vi "AG SubNavUtil.vi"(7 "Progress Ref":refnum<vi>, 8 "error out":errorcluster, 9 "AG SubNav Colors":T1={"On Tab Background"=14869218, "Off Tab Background"=12763842, "Text On Color"=5395026, "Text Off Color"=16777225}, 10 "NewVal":i32, 11 "Tab Ref":refnum<vi>) -> (0 "error IO":errorcluster)   [LabVIEW 2012]
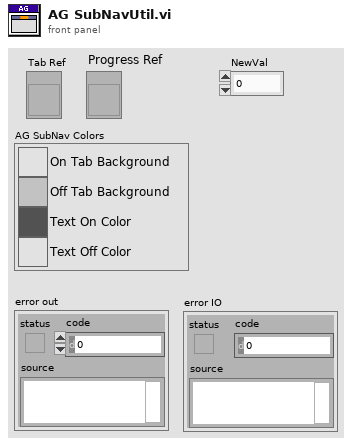
[diagram p1: front panel]
types:
  T1 = cluster{"On Tab Background":u32, "Off Tab Background":u32, "Text On Color":u32, "Text Off Color":u32}
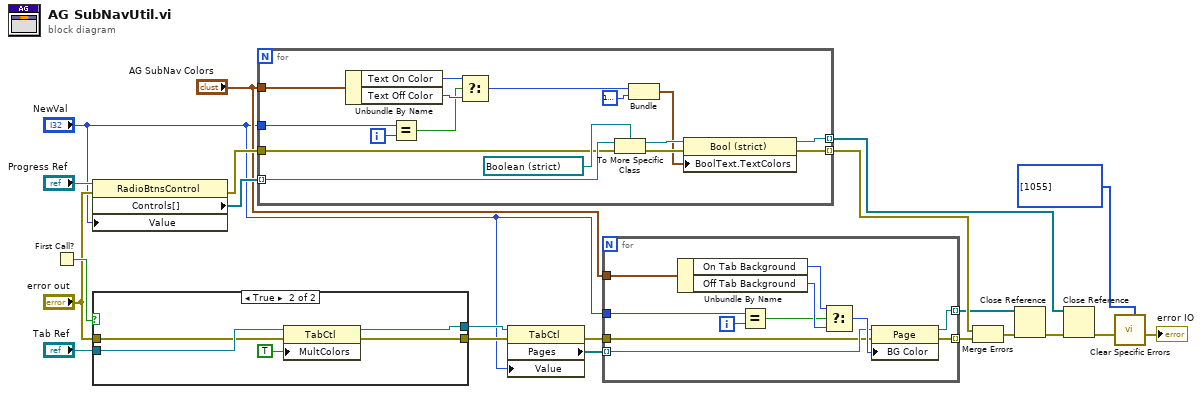
[diagram p0: block diagram]
diagram:
  n1 = First Call?() -> (First Call?: T/F=w20:bool)
  n2 = property class="RadioBtnsControl"(reference="Progress Ref", error in="error out", "Value"="NewVal") -> (error out=w15:errorcluster, "Controls[]"=w16:refnum<vi>[])  [unwired: 1 out]
  n3 = case shown="True" w20 {
    tunnel: "Tab Ref" -> [w22 w28]
    tunnel: "error out" -> [w23 w27]
    tunnel: [w23 w26] -> w19
    tunnel: [w22 w25] -> w18
    frame False {
    }
    frame True {
      n4 = property on="Property Node" class="TabCtl"(reference=w28, error in=w27, "MultColors"=TRUE ("Allow Multiple Colors")) -> (reference out=w25:refnum<vi>, error out=w26:errorcluster)
    }
  }
  n5 = for {
    tunnel: "NewVal" -> [w43]
    tunnel: w16 -> [w39] mode=indexing
    tunnel: "AG SubNav Colors" -> [w40]
    tunnel: w15 -> [w31]
    tunnel: [w30] -> w13 mode=indexing
    tunnel: [w29] -> w9 mode=indexing
    i -> [w44]
    n6 = Unbundle By Name(w40) -> ("Text On Color"=w35:u32, "Text Off Color"=w34:u32)
    n7 = Equal?(x=w43, y=w44) -> (x = y?=w33:bool)
    n8 = Select(t=w35, s=w33, f=w34) -> (s? t:f=w32:u32)
    n9 = To More Specific Class(target class=refnum<vi> refnum ("Radio Selection 1"), reference=w39, error in=w31) -> (specific class reference=w42:refnum<vi>, error out=w38:errorcluster)
    n10 = Bundle("Text Off Color"=w32, u32 16777216) -> (w36:cluster{"Text Off Color":u32, u32})  [unwired: 1 in]
    n11 = property class="Bool (strict)"(reference=w42, error in=w38, "BoolText.TextColors"=w36) -> (reference out=w30:refnum<vi>, error out=w29:errorcluster)
  }
  n12 = property on="Property Node" class="TabCtl"(reference=w18, error in=w19, "Value"="NewVal") -> (error out=w2:errorcluster, "Pages"=w10:refnum<vi>[])  [unwired: 1 out]
  n13 = for {
    tunnel: "AG SubNav Colors" -> [w55]
    tunnel: "NewVal" -> [w53]
    tunnel: w10 -> [w48] mode=indexing
    tunnel: [w47] -> w8 mode=indexing
    tunnel: [w46] -> w6 mode=indexing
    tunnel: w2 -> [w45]
    i -> [w54]
    n14 = Unbundle By Name(w55) -> ("On Tab Background"=w52:u32, "Off Tab Background"=w51:u32)
    n15 = Equal?(x=w53, y=w54) -> (x = y?=w50:bool)
    n16 = Select(t=w52, s=w50, f=w51) -> (s? t:f=w49:u32)
    n17 = property on="Property Node" class="Page"(reference=w48, error in=w45, "BG Color"=w49) -> (reference out=w46:refnum<vi>, error out=w47:errorcluster)
  }
  n18 = Merge Errors(w9, w8) -> (w14:errorcluster)
  n19 = Close Reference(reference=w6, error in (no error)=w14) -> (error out=w12:errorcluster)
  n20 = Close Reference(reference=w13, error in (no error)=w12) -> (error out=w5:errorcluster)
  n21 = call <userlib>:"Clear Specific Errors.vi"("Error Codes"=i32[] [1055], "Error In"=w5) -> ("Error Out"=→"error IO":errorcluster)  [unwired: 8 in, 1 out]
